vi "myRIO Main v2.vi"() -> ()   [LabVIEW 2014]
uses:
  Sensors/IMU - Adafruit BNO055/IMU Control.ctl
  <vilib>/Utility/RT CPU Load.ctl
  Sensors/Time of Flight - VL6180/VL6180 states.ctl
  <vilib>/Platform/TimedLoop/XDataNode/timing_clust.ctl
  <vilib>/Platform/TimedLoop/XDataNode/nitl_modes.ctl
  <vilib>/Platform/TimedLoop/XDataNode/wakeup.ctl
  <vilib>/myRIO/Instrument Drivers/Onboard IO/DIO/typedefs/DIO Reference.ctl
  <vilib>/myRIO/Common/Instrument Driver Framework/Utilities/typedefs/myRIO Generic Hardware Reference.ctl
  <vilib>/myRIO/Common/Instrument Driver Framework/Utilities/typedefs/Hardware Version Enum.ctl
  <vilib>/myRIO/Common/Instrument Driver Framework/Utilities/typedefs/myRIO v1.0 Reference.ctl
  <vilib>/myRIO/Common/Instrument Driver Framework/Utilities/typedefs/Generic FPGA Reference.ctl
  <vilib>/myRIO/Common/Instrument Driver Framework/myRIO v1.0/DIO/typedefs/DIO Channels List.ctl
  <vilib>/myRIO/Common/Instrument Driver Framework/myRIO v1.0/DIO/typedefs/DIO Channels Enum.ctl
  <vilib>/userdefined/High Color/nirio_resource_hc.ctl
  Sensors/Time of Flight - VL6180/VL6180 Resource.ctl
  <vilib>/myRIO/Common/Instrument Driver Framework/Utilities/vis/Is FPGA Ref Available.vi
  <vilib>/myRIO/Common/Instrument Driver Framework/myRIO v1.0/DIO/vis/myRIO v1.1 Open DIO.vi
  <vilib>/myRIO/Instrument Drivers/Onboard IO/DIO/vis/Read.vi
  <vilib>/myRIO/Instrument Drivers/Onboard IO/DIO/vis/Write.vi
  <vilib>/MakerHub/LINX/Public/Peripherals/Digital/Digital Write 1 Chan.vi
  <vilib>/myRIO/Common/Instrument Driver Framework/Utilities/vis/Validate Channels.vi
  <vilib>/myRIO/Common/Instrument Driver Framework/myRIO v1.0/DIO/vis/myRIO v1.0 Reserve DIO.vi
  <vilib>/MakerHub/LINX/Public/Utilities/Check Channel.vi
  <vilib>/MakerHub/LINX/Public/Peripherals/Digital/Digital Write N Chans.vi
  <vilib>/myRIO/Common/Instrument Driver Framework/myRIO v1.0/Resource Manager/vis/myRIO v1.0 Reserve Channel List.vi
  <vilib>/myRIO/Common/Instrument Driver Framework/myRIO v1.0/DIO/vis/myRIO v1.0 Build MUX Configuration DIO.vi
  <vilib>/MakerHub/LINX/Private/Local IO/LinxDigitalWrite.vi
  <vilib>/myRIO/Common/Instrument Driver Framework/myRIO v1.0/Resource Manager/vis/myRIO v1.0 Reserve Channel.vi
  <vilib>/myRIO/Common/Instrument Driver Framework/myRIO v1.0/Resource Manager/vis/myRIO v1.0 Unreserve Channel.vi
  <vilib>/myRIO/Common/Instrument Driver Framework/myRIO v1.0/Resource Manager/vis/myRIO v1.0 Create Configuration List.vi
  <vilib>/MakerHub/LINX/Private/myRIO/Utilities/Get DIO Channel Name.vi
  <vilib>/myRIO/Common/Instrument Driver Framework/myRIO v1.0/Resource Manager/vis/myRIO v1.0 Build Mutex Name.vi
  <vilib>/MakerHub/LINX/Public/Utilities/Open Local.vi
  <vilib>/MakerHub/LINX/Private/Utilties/Generate Error.vi
  <vilib>/MakerHub/LINX/Private/Local IO/LinxI2cOpen.vi
  <vilib>/Utility/VariantDataType/GetNumericInfo.vi
  <vilib>/Utility/error.llb/Error Cluster From Error Code.vi
  <vilib>/myRIO/Common/Instrument Driver Framework/myRIO v1.0/myRIO v1.1 Open.vi
  <vilib>/myRIO/Common/Instrument Driver Framework/Utilities/vis/IO Manager.vi
  <vilib>/myRIO/Common/Instrument Driver Framework/Utilities/vis/Configuration Manager.vi
  <vilib>/myRIO/Common/Instrument Driver Framework/myRIO v1.0/Resource Manager/vis/myRIO v1.0 Configure IO.vi
  <vilib>/myRIO/Common/Instrument Driver Framework/myRIO v1.0/myRIO v1.0 Close.vi
  <vilib>/myRIO/Common/Instrument Driver Framework/myRIO v1.0/DIO/vis/myRIO v1.0 Write DIO.vi
  <vilib>/myRIO/Instrument Drivers/Onboard IO/DIO/vis/Smart Open.vi
  <vilib>/myRIO/Common/Instrument Driver Framework/myRIO v1.0/DIO/vis/myRIO v1.0 Read DIO.vi
  <vilib>/myRIO/Express VI/Onboard IO/DO/DO Express VI.xnode
  <vilib>/myRIO/Instrument Drivers/Onboard IO/DIO/vis/myRIO DIO Open.xnode
  <vilib>/platform/TimedLoop/XDataNode/XDataNode.xnode
  <vilib>/myRIO/Express VI/Onboard IO/DI/DI Express VI.xnode
  <vilib>/MakerHub/LINX/LMH-LINX.lvlib
  <vilib>/Platform/TimedLoop/XDataNode/XDNodeRunTimeDep.lvlib
  <vilib>/myRIO/Instrument Drivers/Onboard IO/DIO/DIO.lvlib
  <vilib>/NI_Real-Time Target Support.lvlib
panel:
  in  "stop":bool
  in  "Enqueue Element":bool
  out "CPU loads":T1[](array[typedef]) {"ISR (%)" format="%#.2f"; "Idle (%)" format="%#.2f"; "Background (%)" format="%#.2f"; "Normal (%)" format="%#.2f"; "Above Normal (%)" format="%#.2f"; "High (%)" format="%#.2g"; "Timed Structures (%)" format="%#.2g"; "Time Critical (%)" format="%#.2g"; "Total (%)" format="%#.2g"}
  out "Pod Health":cluster{"Urgency":u32, "Status":string}
  out "Conversion Time (S)":dbl format="%#_g s"
  out "Power":dbl(knob) scale=0.0..10.0
  out "Current":dbl(knob) scale=0.0..2.0
  out "Voltage":dbl(knob) scale=11.0..12.0
  out "Pressure":i32(graph)
  out "Temp1":dbl(slide) scale=0.0..100.0
  out "V & P Monitor":cluster{"Voltage (Total)":dbl, "Power":dbl}(graph)
  in  "Sensor Power":bool=TRUE
  out "Laser Error":bool
  in  "Reset":bool
  in  "Stop":bool
  in  "Wait (ms)":u32=10
  out "ToF Loop Rate":u32
  in  "Speed Read":bool
  out "Attempts":i32
  out "Sensor Error Code":u8
  in  "Attempts before Timeout":u16=10
  in  "delay":u32=100
  in  "I2C Channel":u8
  out "Sensors Online":bool[](array[boolean])
  in  "# of sensors":i32=5
  out "Status":string
  in  "Track Location":dbl(slide) scale=0.0..5000.0
  out "Structure\nStress":dbl(slide) scale=2.4..2.6
  out "Track Position":T2
  out "Battery (Primary)":dbl(slide) scale=0.0..100.0 scale format="%.1f%"
  out "IMU":T3 {"Gyroscope"."Z" scale=-45.0..45.0; "Gyroscope"."Y" scale=-45.0..45.0; "Gyroscope"."X" scale=-45.0..45.0; "Magnetometer"."Z" scale=-2500.0..2500.0; "Magnetometer"."Y" scale=-2500.0..2500.0; "Magnetometer"."X" scale=-2500.0..2500.0; "Accelerometer"."Z" scale=-5.0..5.0; "Accelerometer"."Y" scale=-5.0..5.0; "Accelerometer"."X" scale=-5.0..5.0}
  out "Gap 4":u8(slide) scale=0.0..100.0
  out "Gap 3":u8(slide) scale=0.0..200.0
  out "Rail Gap 2":u8(slide) scale=0.0..100.0
  out "Gap 2":u8(slide) scale=0.0..100.0
  out "Temp 2":dbl(slide) scale=0.0..100.0
  out "Rail Gap 1":u8(slide) scale=0.0..100.0
  out "Gap 1":u8(slide) scale=0.0..100.0
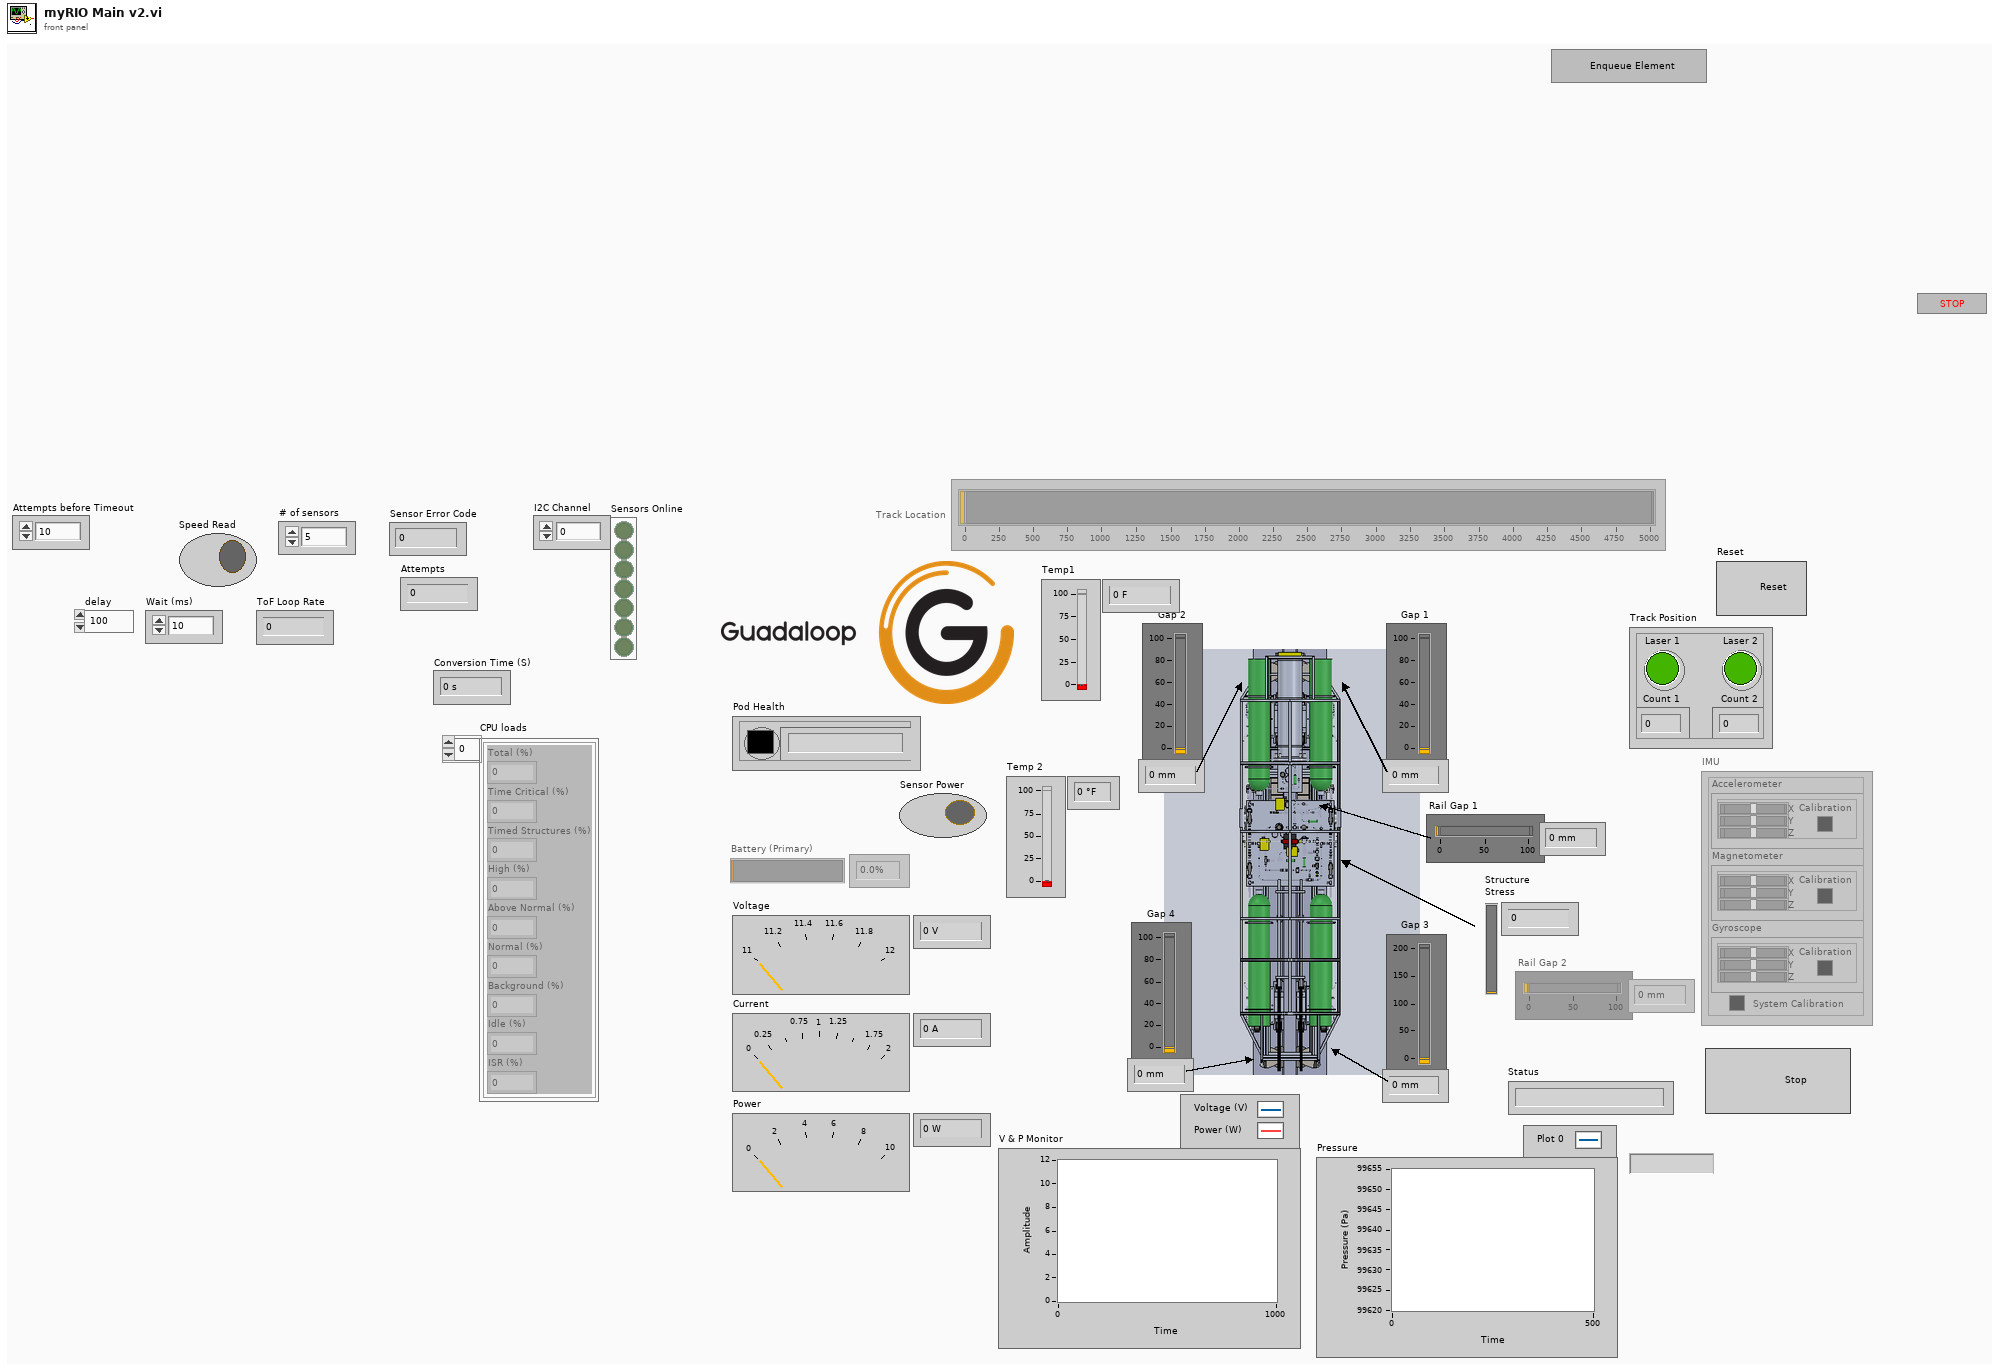
[diagram p1: front panel]
types:
  T1 = typedef "NI_Real-Time Target Support.lvlib/RT CPU Load.ctl" = cluster{"Total (%)":dbl, "Time Critical (%)":dbl, "Timed Structures (%)":dbl, "High (%)":dbl, "Above Normal (%)":dbl, "Normal (%)":dbl, "Background (%)":dbl, "Idle (%)":dbl, "ISR (%)":dbl}
  T2 = cluster{"Laser 1":bool, "Count 1":u32, "Laser 2":bool, "Count 2":u32}
  T3 = typedef "IMU Control.ctl" = cluster{"Accelerometer":cluster{"X":dbl, "Y":dbl, "Z":dbl, "Calibration":u32}, "Magnetometer":cluster{"X":dbl, "Y":dbl, "Z":dbl, "Calibration":u32}, "Gyroscope":cluster{"X":dbl, "Y":dbl, "Z":dbl, "Calibration":u32}, "System Calibration":u32}
  T4 = typedef "VL6180 states.ctl" = enum16{"Ping All", "Initialize", "Read"}
  T5 = typedef "LMH-LINX.lvlib/LINX Ref.ctl" = cluster{"IO":T6, "Interface":T7, "LINX Device Config":T8}
  T6 = typedef "LMH-LINX.lvlib/Platform.ctl" = enum16{"Remote", "Local"}
  T7 = typedef "LMH-LINX.lvlib/Interface.ctl" = enum16{"Serial", "TCP"}
  T8 = typedef "LMH-LINX.lvlib/Device.lvlib/LINX Device Config.ctl" = cluster{"Interface":T7, "COM Port":refnum<visa-resource-name>, "TCP Configuration":T9, "Device Family":u8, "Device ID":u8, "Device Name":string, "TCP Ref":refnum<k5>, "Channels":T10}
  T9 = typedef "LMH-LINX.lvlib/Device.lvlib/TCP Config.ctl" = cluster{"IP Address":string, "Port":u16}
  T10 = typedef "LMH-LINX.lvlib/Channels.ctl" = cluster{"DI":u8[], "DO":u8[], "AI":u8[], "AO":u8[], "PWM":u8[], "QE":u8[], "UART":u8[], "I2C 2":u8[], "SPI":u8[], "CAN":u8[], "Servo":u8[], "AI Ref (V)":dbl, "AI Resolution (Bits)":u8, "AO Ref (V)":dbl, "AO Resolution (Bits)":u8}
  T11 = typedef "XDNodeRunTimeDep.lvlib/timing_clust.ctl" = cluster{"Expected End [f-1]":u64, "Actual End [f-1]":u64, "Finished Late? [f-1]":bool, "Expected End [i-1]":u64, "Actual End [i-1]":u64, "Finished Late? [i-1]":bool, "Expected Start [i]":u64, "Actual Start [i]":u64, "Expected Start [f]":u64, "Actual Start [f]":u64, "Source Name":string, "Structure Name":string, "Period":i64, "Deadline":i64, "Offset":i64, "Start":i64, "Priority":i32, "Timeout":i32, "Mode":T12, "Wakeup Reason":T13, "Error":errorcluster, "Source Type":string, "Secondary Source Type":string, "Global End Time":u64, "Global Start Time":u64, "Frame Duration":u64, "Iteration Duration":u64, "Assigned CPU":i32, "I/O Scan Engine Mode":u32}
  T12 = typedef "XDNodeRunTimeDep.lvlib/nitl_modes.ctl" = enum32{"No Change", "Process missed periods, maintain original phase", "Discard missed periods, maintain original phase", "Process missed periods, ignore original phase", "Discard missed periods, ignore original phase"}
  T13 = typedef "XDNodeRunTimeDep.lvlib/wakeup.ctl" = enum32{"Normal", "Aborted", "Asynchronous wakeup", "Timing source error", "Timed loop error", "Timeout"}
  T14 = typedef "DIO.lvlib/DIO Reference.ctl" = cluster{"myRIO Reference":T15, "DIO Channels List":T19}
  T15 = typedef "myRIO Generic Hardware Reference.ctl" = cluster{"myRIO Model":T16, "myRIO Hardware Reference":T17}
  T16 = typedef "Hardware Version Enum.ctl" = enum16{"Unknown", "myRIO-1900", "myRIO-1950"}
  T17 = typedef "myRIO v1.0 Reference.ctl" = cluster{"Generic FPGA Reference":T18, "Allow multiple opens":bool}
  T18 = typedef "Generic FPGA Reference.ctl" = refnum<k20>
  T19 = typedef "DIO Channels List.ctl" = T20[]
  T20 = typedef "DIO Channels Enum.ctl" = enum16{"Not Connected", "C/DIO0", "C/DIO1", "C/DIO2", "C/DIO3", "C/DIO4", "C/DIO5", "C/DIO6", "C/DIO7", "A/DIO0", "A/DIO1", "A/DIO2", "A/DIO3", "A/DIO4", "A/DIO5", "A/DIO6", "A/DIO7", "A/DIO8", "A/DIO9", "A/DIO10", "A/DIO11", "A/DIO12", "A/DIO13", "A/DIO14", "A/DIO15", "B/DIO0", "B/DIO1", "B/DIO2", "B/DIO3", "B/DIO4", "B/DIO5", "B/DIO6", "B/DIO7", "B/DIO8", "B/DIO9", "B/DIO10", "B/DIO11", "B/DIO12", "B/DIO13", "B/DIO14", "B/DIO15", "LED0", "LED1", "LED2", "LED3", "Button0"}
  T21 = typedef "nirio_resource_hc.ctl" = tag
  T22 = typedef "VL6180 Resource.ctl" = cluster{"I2C Channel":u8, "I2C Slave Address":u8, "Online":bool}
  T23 = cluster{"Object Temp (°C)":dbl, "Object Temp (°F)":dbl, "Ambient Temp (°C)":dbl, "Ambient Temp (°F)":dbl}
  T24 = typedef "INA219 Measurements.ctl" = cluster{"Voltage (Total)":dbl, "Bus Voltage":dbl, "Shunt Voltage":dbl, "Power":dbl, "Current":dbl}
  T25 = typedef "INA219 Config Options.ctl" = cluster{"I2C":cluster{"Slave Address":u8, "Channel":u8}, "Reset bit":u8, "Bus Voltage Range":u8, "PGA/Shunt Voltage Gain":u8, "Bus Voltage ADC Settings":u8, "Shunt Voltage ADC Settings":u8, "Mode":u8, "Calibration Value":u16}
  T26 = typedef "BMP180 Config Options.ctl" = cluster{"I2C":cluster{"Slave Address":u8, "Channel":u8}, "Mode":enum8{"Ultra Low Power", "Standard", "High Resolution", "Ultra High Resolution"}, "Cal Coefs":cluster{"AC1":cluster{"Addr:":u8, "Val:":u16}, "AC2":cluster{"Addr:":u8, "Val:":u16}, "AC3":cluster{"Addr:":u8, "Val:":u16}, "AC4":cluster{"Addr:":u8, "Val:":u16}, "AC5":cluster{"Addr:":u8, "Val:":u16}, "AC6":cluster{"Addr:":u8, "Val:":u16}, "B1":cluster{"Addr:":u8, "Val:":u16}, "B2":cluster{"Addr:":u8, "Val:":u16}, "MB":cluster{"Addr:":u8, "Val:":u16}, "MC":cluster{"Addr:":u8, "Val:":u16}, "MD":cluster{"Addr:":u8, "Val:":u16}}}
  T27 = typedef "ADS1015 Config Options.ctl" = cluster{"I2C":cluster{"Slave Address":u8, "Channel":u8}, "ADC":cluster{"Channel":u8, "Expected Range (Programmable Gain Amplifier)":u8, "Sampling Mode":u8, "Sampling Rate":u8, "Comparator Mode":u8, "Comparator Polarity":u8, "Latching Comparator":u8, "Comparator Queue & Disable":u8}}
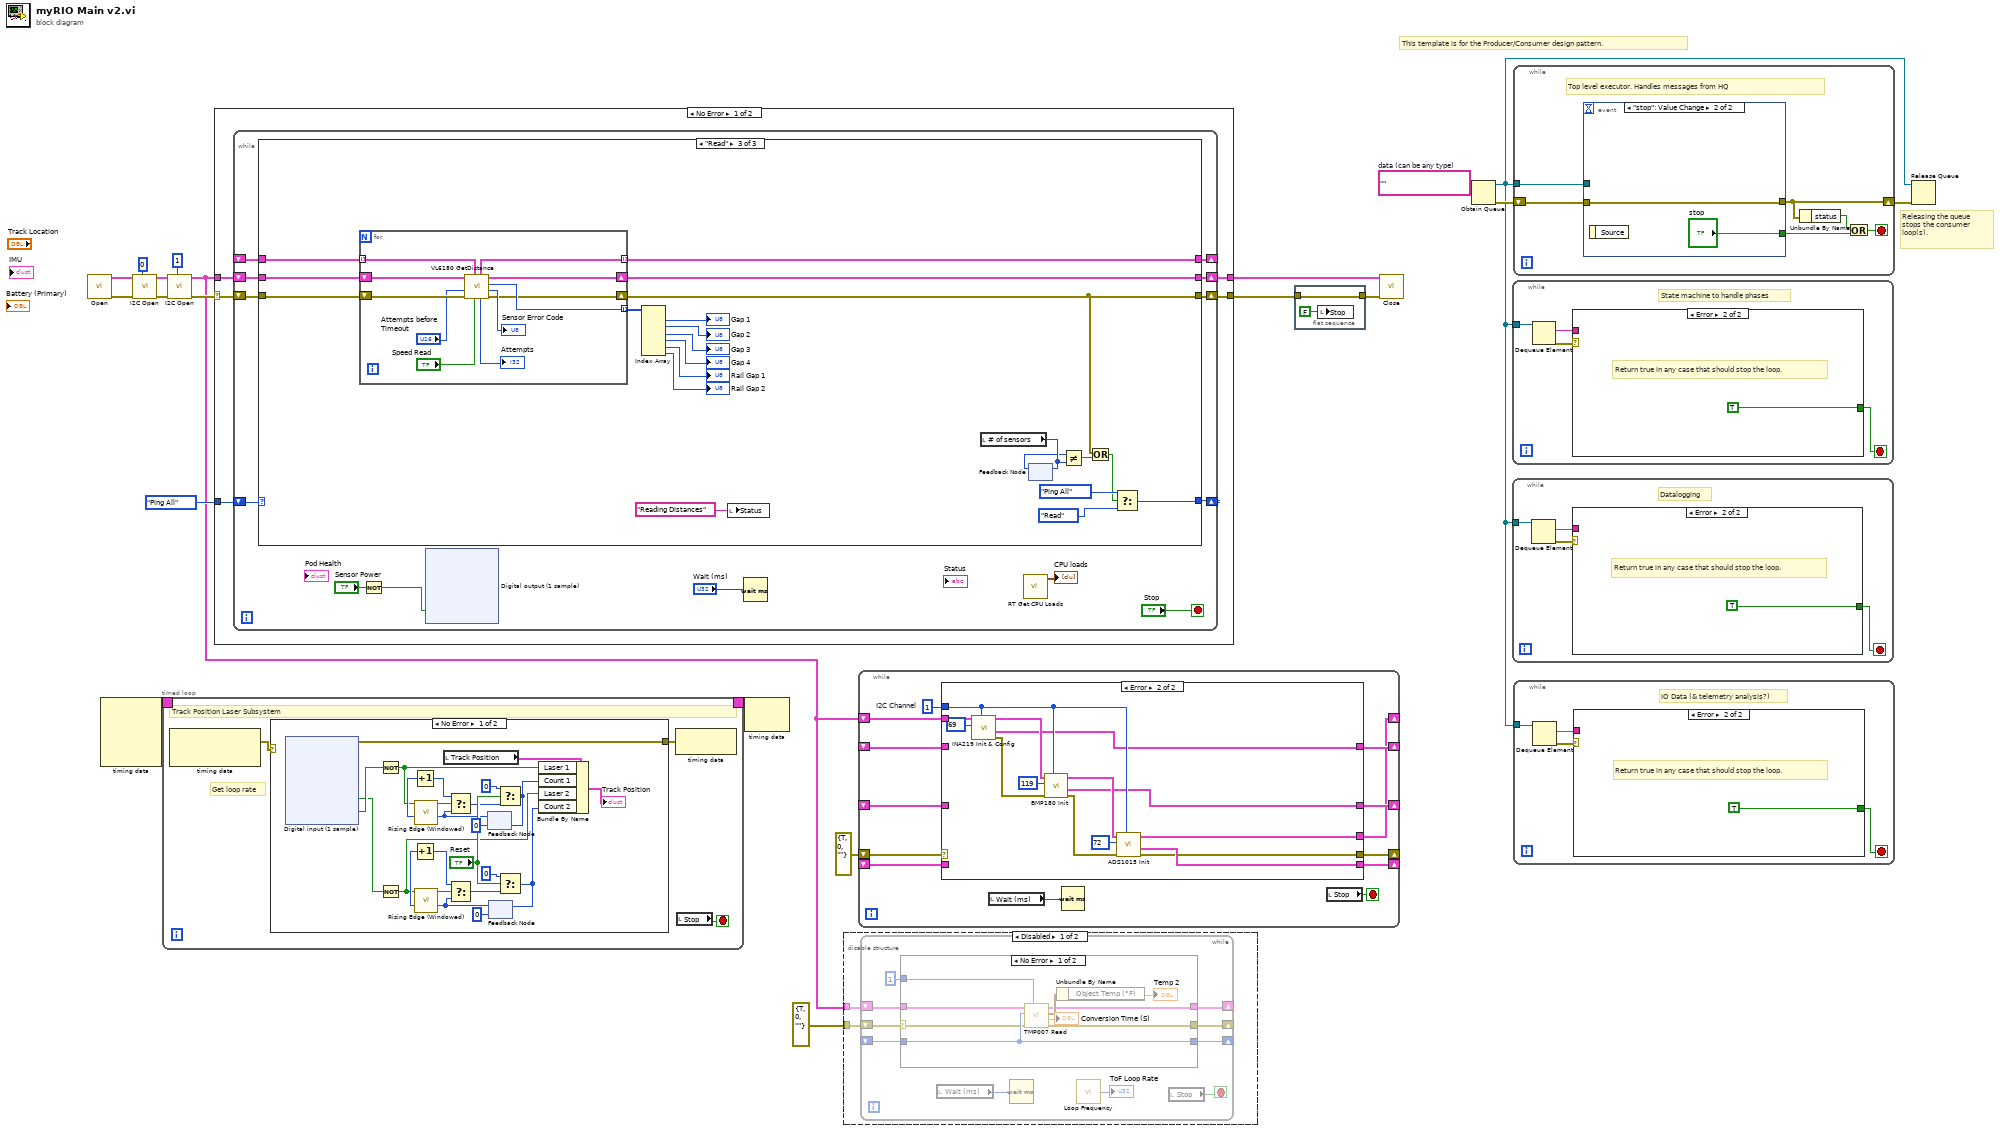
[diagram p0: block diagram]
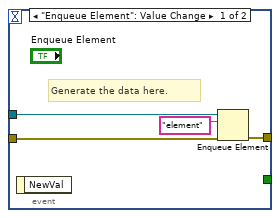
[diagram p5: hidden frame]
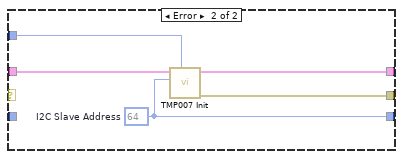
[diagram p6: hidden frame]
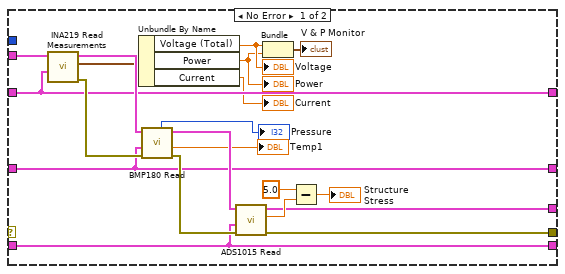
[diagram p8: hidden frame]
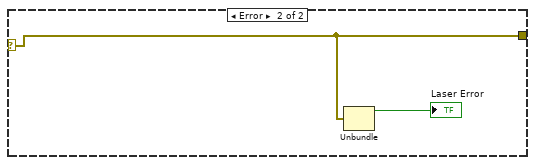
[diagram p9: hidden frame]
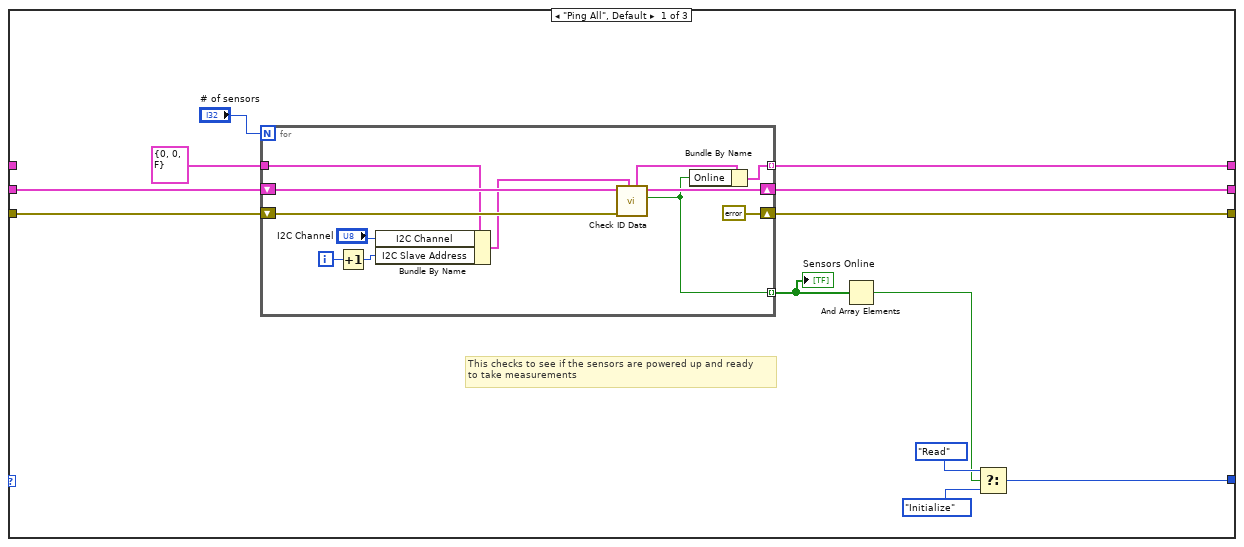
[diagram p10: hidden frame]
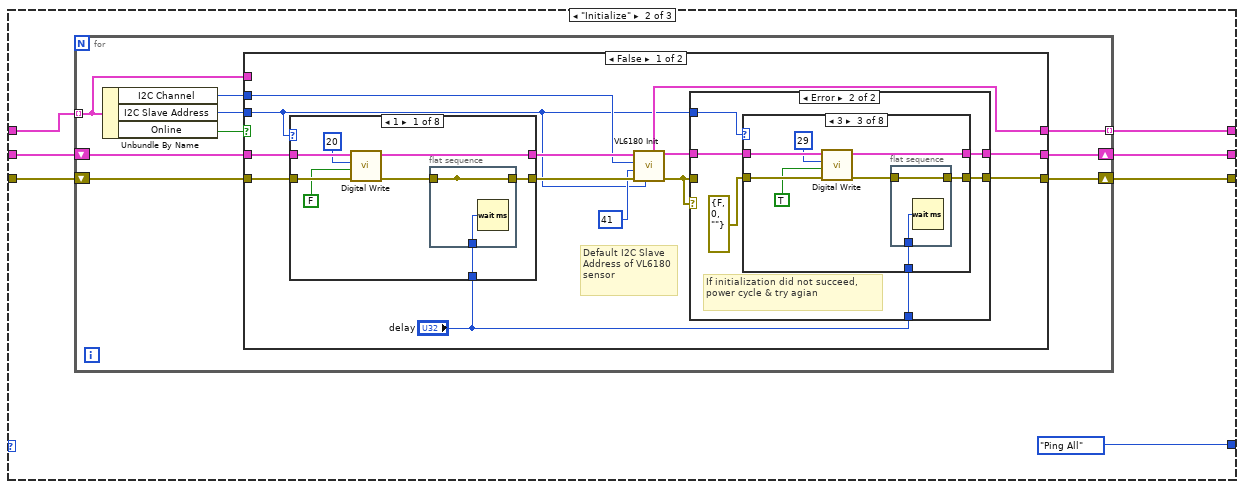
[diagram p11: hidden frame]
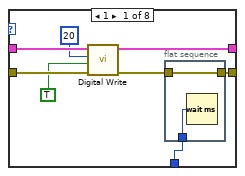
[diagram p13: hidden frame]
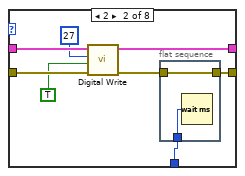
[diagram p14: hidden frame]
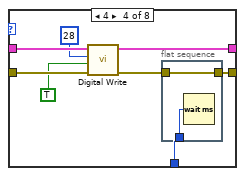
[diagram p15: hidden frame]
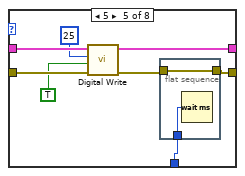
[diagram p16: hidden frame]
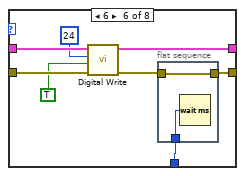
[diagram p17: hidden frame]
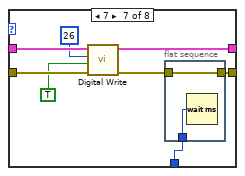
[diagram p18: hidden frame]
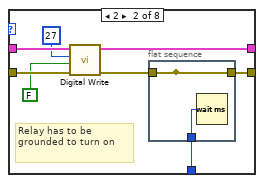
[diagram p20: hidden frame]
diagram:
  w2 = ""  # data (can be any type)
  # "Releasing the queue stops the consumer loop(s)."
  # "This template is for the Producer/Consumer design pattern."
  n1 = call-poly <vilib>:"Open.vi"() -> ("Error Out"=w10:errorcluster, "LINX Resource"=w11:T5)  [unwired: 9 in, 1 out]
  n2 = node-c288() -> (w16:T11)  [unwired: 4 in]
  n3 = call <vilib>:"I2C Open.vi"("I2C Channel (0)"=u8 0, "Error In"=w10, "LINX Resource"=w11) -> ("Error Out"=w9:errorcluster, "LINX Resource"=w8:T5)  [unwired: 7 in]
  n4 = timed-loop {
    timing: w16 -> [_]
    timing-out: [_] -> w15
    stop <- w23 stop-if-true
    # "Get loop rate"
    # "Track Position Laser Subsystem"
    n5 = node-c288() -> (w22:errorcluster)  [unwired: 1 in, 1 out]
    n6 = case shown="No Error" w22 {
      selector: w22 -> [_ w83]
      tunnel: [w28 w83] -> w21
      frame No Error {
        n7 = xnode "Digital input (1 sample)"() -> ("Laser 1 (A/DIO0 (Pin 11))"=w24:bool, "Laser 2 (A/DIO1 (Pin 13))"=w25:bool, "error out"=w28:errorcluster)  [unwired: 1 in]
        n8 = Not(x=w25) -> (.not. x?=w33:bool)
        n9 = Not(x=w24) -> (.not. x?=w30:bool)
        n10 = call "Rising Edge (Windowed).vi"("Input"=w33) -> ("Rising Edge?"=w38:bool)  [unwired: 10 in]
        n11 = call "Rising Edge (Windowed).vi"("Input"=w30) -> ("Rising Edge?"=w31:bool)  [unwired: 10 in]
        n12 = local read "Track Position"() -> (w35:T2)
        n13 = feedback #1(u32 0 ("t")) -> (w37:u32)
        n14 = Increment(x=w37) -> (x+1=w39:u32)
        n15 = Select(t=w39, s=w38, f=w37) -> (s? t:f=w40:u32)
        n16 = feedback #2(u32 0 ("t")) -> (w36:u32)
        n17 = Increment(x=w36) -> (x+1=w42:u32)
        n18 = Select(t=w42, s=w31, f=w36) -> (s? t:f=w43:u32)
        n19 = Select(t=u32 0, s="Reset", f=w40) -> (s? t:f=w32:u32)
        n20 = feedback-in #1(w32) -> ()
        n21 = Select(t=u32 0, s="Reset", f=w43) -> (s? t:f=w29:u32)
        n22 = feedback-in #2(w29) -> ()
        n23 = Bundle By Name(cluster=w35, "Laser 1"=w33, "Count 1"=w32, "Laser 2"=w30, "Count 2"=w29) -> (→"Track Position":T2)
      }
      frame Error {
        n24 = Unbundle(w83) -> ("status"=→"Laser Error":bool)  [unwired: 2 out]
      }
    }
    n25 = node-c288(w21) -> ()  [unwired: 1 out]
    n26 = local read "Stop"() -> (w23:bool)
  }
  n27 = call <vilib>:"I2C Open.vi"("I2C Channel (0)"=u8 1, "Error In"=w9, "LINX Resource"=w8) -> ("Error Out"=w14:errorcluster, "LINX Resource"=w5:T5)  [unwired: 7 in]
  n28 = case shown="No Error" w14 {
    selector: w14 -> [w91 w384]
    tunnel: [w93 w384] -> w18
    tunnel: [w92 w383] -> w19
    tunnel: VL6180_states."Ping All" -> [w90 _]
    tunnel: w5 -> [w89 w383]
    frame No Error {
      n29 = while {
        shift-right: [w98] -> w92
        shift-left: w89 -> [w104]
        shift-right: [w97] -> w93
        shift-left: w91 -> [w103]
        shift-right: [w99] -> _
        shift-left: _ -> [w102]
        shift-right: [w100] -> _
        shift-left: w90 -> [w101]
        stop <- "Stop" stop-if-true
        n30 = case shown="\"Read\"" w101 {
          tunnel: w104 -> [w118 w137 w334]
          tunnel: w103 -> [w117 w131 w336]
          tunnel: w102 -> [_ w135 w333]
          tunnel: [w115 w132 w335] -> w99
          tunnel: [w116 w134 w328] -> w98
          tunnel: [w114 VL6180_states."Ping All" w332] -> w100
          tunnel: [w113 w133 w327] -> w97
          frame "Ping All", Default {
            # "This checks to see if the sensors are powered up and ready\nto take measurements"
            n31 = for {
              N: "# of sensors" -> [_]
              tunnel: T22 {"I2C Channel"=0, "I2C Slave Address"=0, "Online"=FALSE} ("VL6180 Resource out") -> [w123]
              shift-right: [w126] -> w116
              shift-left: w118 -> [w130]
              tunnel: [w125] -> w115 mode=indexing
              tunnel: [w124] -> w112 mode=indexing
              shift-right: [errorcluster {"status"=FALSE, "code"=0, "source"=""} ("error IO")] -> w113
              shift-left: w117 -> [w129]
              i -> [w127]
              n32 = Increment(x=w127) -> (x+1=w120:i32)
              n33 = Bundle By Name(cluster=w123, "I2C Channel"="I2C Channel", "I2C Slave Address"=w120) -> (w122:T22)
              n34 = call "Check ID Data.vi"("VL6180 Resource"=w122, "Error In"=w129, "LINX Resource"=w130) -> ("Same Model?"=w124:bool, "LINX Resource"=w126:T5, "VL6180 Resource"=w128:T22)  [unwired: 5 in, 1 out]
              n35 = Bundle By Name(cluster=w128, "Online"=w124) -> (w125:T22)
            }
            "Sensors Online" <- w112
            n36 = And Array Elements(Boolean array=w112) -> (logical AND=w109:bool)
            n37 = Select(t=VL6180_states."Read", s=w109, f=VL6180_states."Initialize") -> (s? t:f=w114:T4)
          }
          frame "Initialize" {
            n38 = for {
              tunnel: w135 -> [w138] mode=indexing
              shift-right: [w145] -> w134
              shift-left: w137 -> [w146]
              shift-right: [w144] -> w133
              shift-left: w131 -> [w140]
              tunnel: [w141] -> w132 mode=indexing
              n39 = Unbundle By Name(w138) -> ("I2C Channel"=w143:u8, "I2C Slave Address"=w142:u8, "Online"=w139:bool)
              n40 = case shown="False" w139 {
                tunnel: w146 -> [w159 w315]
                tunnel: w140 -> [w156 w314]
                tunnel: [w153 w315] -> w145
                tunnel: [w152 w314] -> w144
                tunnel: w143 -> [w148 _]
                tunnel: w142 -> [w147 _]
                tunnel: [w154 w313] -> w141
                tunnel: w138 -> [_ w313]
                frame False {
                  # "Default I2C Slave Address of VL6180 sensor"
                  n41 = case shown="1" w147 {
                    tunnel: w159 -> [w247 w257 w267 w277 w287 w297 w307 w311]
                    tunnel: [w246 w256 w266 w276 w286 w296 w306 w311] -> w158
                    tunnel: [w242 w252 w261 w271 w281 w291 w301 w310] -> w157
                    tunnel: w156 -> [w245 w255 w265 w275 w285 w295 w305 w310]
                    tunnel: "delay" -> [w240 w250 w260 w270 w280 w290 w300 _]
                    frame 1 {
                      n42 = call-poly <vilib>:"Digital Write.vi"("Error In"=w245, "Output Value"=FALSE, "DO Channel"=u8 20, "LINX Resource"=w247) -> ("Error Out"=w241:errorcluster, "LINX Resource"=w246:T5)  [unwired: 6 in]
                      n43 = flat-sequence {
                        tunnel: [w249] -> _
                        tunnel: [w249] -> w242
                        tunnel: w241 -> [w249]
                        tunnel: w240 -> [w248]
                        frame #0 {
                          n44 = Wait (ms)(milliseconds to wait=w248) -> ()  [unwired: 1 out]
                        }
                      }
                    }
                    frame 2 {
                      # "Relay has to be grounded to turn on"
                      n45 = call-poly <vilib>:"Digital Write.vi"("Error In"=w255, "Output Value"=FALSE, "DO Channel"=u8 27, "LINX Resource"=w257) -> ("Error Out"=w251:errorcluster, "LINX Resource"=w256:T5)  [unwired: 6 in]
                      n46 = flat-sequence {
                        tunnel: [w259] -> _
                        tunnel: [w259] -> w252
                        tunnel: w251 -> [w259]
                        tunnel: w250 -> [w258]
                        frame #0 {
                          n47 = Wait (ms)(milliseconds to wait=w258) -> ()  [unwired: 1 out]
                        }
                      }
                    }
                    frame 3 {
                      n48 = call-poly <vilib>:"Digital Write.vi"("Error In"=w265, "Output Value"=FALSE, "DO Channel"=u8 29, "LINX Resource"=w267) -> ("Error Out"=w262:errorcluster, "LINX Resource"=w266:T5)  [unwired: 6 in]
                      n49 = flat-sequence {
                        tunnel: w262 -> [w269]
                        tunnel: [w269] -> w261
                        tunnel: w260 -> [w268]
                        frame #0 {
                          n50 = Wait (ms)(milliseconds to wait=w268) -> ()  [unwired: 1 out]
                        }
                      }
                    }
                    frame 4 {
                      n51 = call-poly <vilib>:"Digital Write.vi"("Error In"=w275, "Output Value"=FALSE, "DO Channel"=u8 28, "LINX Resource"=w277) -> ("Error Out"=w272:errorcluster, "LINX Resource"=w276:T5)  [unwired: 6 in]
                      n52 = flat-sequence {
                        tunnel: w272 -> [w279]
                        tunnel: [w279] -> w271
                        tunnel: w270 -> [w278]
                        frame #0 {
                          n53 = Wait (ms)(milliseconds to wait=w278) -> ()  [unwired: 1 out]
                        }
                      }
                    }
                    frame 5 {
                      n54 = call-poly <vilib>:"Digital Write.vi"("Error In"=w285, "Output Value"=FALSE, "DO Channel"=u8 25, "LINX Resource"=w287) -> ("Error Out"=w282:errorcluster, "LINX Resource"=w286:T5)  [unwired: 6 in]
                      n55 = flat-sequence {
                        tunnel: w282 -> [w289]
                        tunnel: [w289] -> w281
                        tunnel: w280 -> [w288]
                        frame #0 {
                          n56 = Wait (ms)(milliseconds to wait=w288) -> ()  [unwired: 1 out]
                        }
                      }
                    }
                    frame 6 {
                      n57 = call-poly <vilib>:"Digital Write.vi"("Error In"=w295, "Output Value"=FALSE, "DO Channel"=u8 24, "LINX Resource"=w297) -> ("Error Out"=w292:errorcluster, "LINX Resource"=w296:T5)  [unwired: 6 in]
                      n58 = flat-sequence {
                        tunnel: w292 -> [w299]
                        tunnel: [w299] -> w291
                        tunnel: w290 -> [w298]
                        frame #0 {
                          n59 = Wait (ms)(milliseconds to wait=w298) -> ()  [unwired: 1 out]
                        }
                      }
                    }
                    frame 7 {
                      n60 = call-poly <vilib>:"Digital Write.vi"("Error In"=w305, "Output Value"=FALSE, "DO Channel"=u8 30, "LINX Resource"=w307) -> ("Error Out"=w302:errorcluster, "LINX Resource"=w306:T5)  [unwired: 6 in]
                      n61 = flat-sequence {
                        tunnel: w302 -> [w309]
                        tunnel: [w309] -> w301
                        tunnel: w300 -> [w308]
                        frame #0 {
                          n62 = Wait (ms)(milliseconds to wait=w308) -> ()  [unwired: 1 out]
                        }
                      }
                    }
                    frame 9, Default {
                      n63 = local write "Status"("Plug new sensor in" ("message")) -> ()
                    }
                  }
                  n64 = call "VL6180 Init.vi"("Change Slave Address"=w147, "Error In"=w157, "I2C Slave Address"=u8 41 ("I2C Slave Address (0)"), "I2C Channel"=w148, "LINX Resource"=w158) -> ("Error Out"=w150:errorcluster, "LINX Resource"=w151:T5, "VL6180 Resource"=w154:T22)  [unwired: 4 in]
                  n65 = case shown="Error" w150 {
                    tunnel: [w161 w167] -> w153
                    tunnel: [w160 w164] -> w152
                    tunnel: w151 -> [w161 w166]
                    tunnel: w150 -> [w160 _]
                    tunnel: "delay" -> [_ w163]
                    tunnel: w147 -> [_ w162]
                    frame No Error {
                      # "Initialization successful"
                    }
                    frame Error {
                      # "If initialization did not succeed, power cycle & try agian"
                      n66 = case shown="3" w162 {
                        tunnel: w166 -> [w175 w185 w195 w205 w215 w225 w235 w239]
                        tunnel: [w174 w184 w194 w204 w214 w224 w234 w239] -> w167
                        tunnel: [w169 w178 w189 w199 w209 w219 w229 w238] -> w164
                        tunnel: errorcluster {"status"=FALSE, "code"=0, "source"=""} ("Error Out") -> [w173 w183 w193 w203 w213 w223 w233 w238]
                        tunnel: w163 -> [w168 w179 w188 w198 w208 w218 w228 _]
                        frame 1 {
                          n67 = call-poly <vilib>:"Digital Write.vi"("Error In"=w173, "Output Value"=TRUE, "DO Channel"=u8 20, "LINX Resource"=w175) -> ("Error Out"=w170:errorcluster, "LINX Resource"=w174:T5)  [unwired: 6 in]
                          n68 = flat-sequence {
                            tunnel: [w177] -> w169
                            tunnel: w170 -> [w177]
                            tunnel: w168 -> [w176]
                            frame #0 {
                              n69 = Wait (ms)(milliseconds to wait=w176) -> ()  [unwired: 1 out]
                            }
                          }
                        }
                        frame 2 {
                          n70 = call-poly <vilib>:"Digital Write.vi"("Error In"=w183, "Output Value"=TRUE, "DO Channel"=u8 27, "LINX Resource"=w185) -> ("Error Out"=w180:errorcluster, "LINX Resource"=w184:T5)  [unwired: 6 in]
                          n71 = flat-sequence {
                            tunnel: [w187] -> w178
                            tunnel: w180 -> [w187]
                            tunnel: w179 -> [w186]
                            frame #0 {
                              n72 = Wait (ms)(milliseconds to wait=w186) -> ()  [unwired: 1 out]
                            }
                          }
                        }
                        frame 3 {
                          n73 = call-poly <vilib>:"Digital Write.vi"("Error In"=w193, "Output Value"=TRUE, "DO Channel"=u8 29, "LINX Resource"=w195) -> ("Error Out"=w190:errorcluster, "LINX Resource"=w194:T5)  [unwired: 6 in]
                          n74 = flat-sequence {
                            tunnel: [w197] -> w189
                            tunnel: w190 -> [w197]
                            tunnel: w188 -> [w196]
                            frame #0 {
                              n75 = Wait (ms)(milliseconds to wait=w196) -> ()  [unwired: 1 out]
                            }
                          }
                        }
                        frame 4 {
                          n76 = call-poly <vilib>:"Digital Write.vi"("Error In"=w203, "Output Value"=TRUE, "DO Channel"=u8 28, "LINX Resource"=w205) -> ("Error Out"=w200:errorcluster, "LINX Resource"=w204:T5)  [unwired: 6 in]
                          n77 = flat-sequence {
                            tunnel: [w207] -> w199
                            tunnel: w200 -> [w207]
                            tunnel: w198 -> [w206]
                            frame #0 {
                              n78 = Wait (ms)(milliseconds to wait=w206) -> ()  [unwired: 1 out]
                            }
                          }
                        }
                        frame 5 {
                          n79 = call-poly <vilib>:"Digital Write.vi"("Error In"=w213, "Output Value"=TRUE, "DO Channel"=u8 25, "LINX Resource"=w215) -> ("Error Out"=w210:errorcluster, "LINX Resource"=w214:T5)  [unwired: 6 in]
                          n80 = flat-sequence {
                            tunnel: [w217] -> w209
                            tunnel: w210 -> [w217]
                            tunnel: w208 -> [w216]
                            frame #0 {
                              n81 = Wait (ms)(milliseconds to wait=w216) -> ()  [unwired: 1 out]
                            }
                          }
                        }
                        frame 6 {
                          n82 = call-poly <vilib>:"Digital Write.vi"("Error In"=w223, "Output Value"=TRUE, "DO Channel"=u8 24, "LINX Resource"=w225) -> ("Error Out"=w220:errorcluster, "LINX Resource"=w224:T5)  [unwired: 6 in]
                          n83 = flat-sequence {
                            tunnel: [w227] -> w219
                            tunnel: w220 -> [w227]
                            tunnel: w218 -> [w226]
                            frame #0 {
                              n84 = Wait (ms)(milliseconds to wait=w226) -> ()  [unwired: 1 out]
                            }
                          }
                        }
                        frame 7 {
                          n85 = call-poly <vilib>:"Digital Write.vi"("Error In"=w233, "Output Value"=TRUE, "DO Channel"=u8 26, "LINX Resource"=w235) -> ("Error Out"=w230:errorcluster, "LINX Resource"=w234:T5)  [unwired: 6 in]
                          n86 = flat-sequence {
                            tunnel: [w237] -> w229
                            tunnel: w230 -> [w237]
                            tunnel: w228 -> [w236]
                            frame #0 {
                              n87 = Wait (ms)(milliseconds to wait=w236) -> ()  [unwired: 1 out]
                            }
                          }
                        }
                        frame 9, Default {
                        }
                      }
                    }
                  }
                }
                frame True {
                }
              }
            }
          }
          frame "Read" {
            n88 = for {
              tunnel: [w343] -> w335 mode=indexing
              shift-right: [w341] -> w328
              shift-left: w334 -> [w342]
              tunnel: w333 -> [w337] mode=indexing
              tunnel: [w340] -> w321 mode=indexing
              shift-right: [w339] -> w327
              shift-left: w336 -> [w347]
              n89 = call "VL6180 GetDistance.vi"("Speed Read"="Speed Read", "VL6180 Resource in"=w337, "error in (no error)"=w347, "Attempts before Timeout"="Attempts before Timeout", "LINX Resource"=w342) -> ("error out"=w339:errorcluster, "Sensor Error Code"=→"Sensor Error Code":u8, "Distance (mm)"=w340:u8, "LINX Resource"=w341:T5, "Attempts"=→"Attempts":i32, "VL6180 Resource out"=w343:T22)  [unwired: 1 in]
            }
            n90 = Index Array(array=w321) -> (element #1=→"Gap 1":u8, element #2=→"Gap 2":u8, element #3=→"Gap 3":u8, element #4=→"Gap 4":u8, element #5=→"Rail Gap 1":u8, element #6=→"Rail Gap 2":u8)  [unwired: 6 in]
            n91 = local write "Status"("Reading Distances" ("Status")) -> ()
            n92 = local read "# of sensors"() -> (w325:i32)
            n93 = feedback-in #3(w325) -> ()
            n94 = feedback #3() -> (w324:i32)  [unwired: 1 in]
            n95 = Not Equal?(x=w324, y=w325) -> (x != y?=w326:bool)
            n96 = Or(x=w327, y=w326) -> (x .or. y?=w323:bool)
            n97 = Select(t=VL6180_states."Ping All", s=w323, f=VL6180_states."Read") -> (s? t:f=w332:T4)
          }
        }
        n98 = Not(x="Sensor Power") -> (.not. x?=w95:bool)
        n99 = xnode "Digital output (1 sample)"("Sens. Pow. (B/DIO7 (Pin 25))"=w95) -> ()  [unwired: 1 in, 1 out]
        n100 = Wait (ms)(milliseconds to wait="Wait (ms)") -> ()  [unwired: 1 out]
        n101 = call <vilib>:"RT Get CPU Loads.vi"() -> ("CPU loads"=→"CPU loads":T1[])  [unwired: 10 in, 1 out]
      }
    }
    frame Error {
    }
  }
  n102 = node-c288(w15) -> ()  [unwired: 1 out]
  n103 = disable-structure shown="Disabled" {
    disable-tunnel: errorcluster {"status"=TRUE, "code"=0, "source"=""} ("error out") -> [w386 _]
    disable-tunnel: w5 -> [w385 _]
    frame Disabled {
      n104 = while {
        shift-right: [w395] -> _
        shift-left: w386 -> [w394]
        shift-right: [w393] -> _
        shift-left: _ -> [w392]
        shift-right: [w389] -> _
        shift-left: w385 -> [w388]
        stop <- w396 stop-if-true
        n105 = case shown="No Error" w394 {
          selector: w394 -> [w399 _]
          tunnel: u8 1 ("I2C Channel") -> [w401 w407]
          tunnel: [w405 w410] -> w395
          tunnel: [w404 w409] -> w393
          tunnel: w392 -> [w404 _]
          tunnel: [w402 w408] -> w389
          tunnel: w388 -> [w398 w406]
          frame No Error {
            n106 = call "TMP007 Read.vi"("I2C Channel"=w401, "error in (no error)"=w399, "I2C Slave Address"=w404, "LINX Resource in"=w398) -> ("error out"=w405:errorcluster, "Conversion Time (S)"=→"Conversion Time (S)":dbl, "Temp Readings"=w403:T23, "LINX Resource"=w402:T5)  [unwired: 4 in]
            n107 = Unbundle By Name(w403) -> ("Object Temp (°F)"=→"Temp 2":dbl)
          }
          frame Error {
            w409 = u8 64  # I2C Slave Address
            n108 = call "TMP007 Init.vi"("I2C Channel"=w407, "I2C Slave Address"=w409, "LINX Resource in"=w406) -> ("error out"=w410:errorcluster, "LINX Resource out"=w408:T5)  [unwired: 7 in]
          }
        }
        n109 = local read "Wait (ms)"() -> (w391:u32)
        n110 = Wait (ms)(milliseconds to wait=w391) -> ()  [unwired: 1 out]
        n111 = call <vilib>:"Loop Frequency.vi"() -> ("Loop Rate (Hz)"=→"ToF Loop Rate":u32)
        n112 = local read "Stop"() -> (w396:bool)
      }
    }
    frame Enabled {
    }
  }
  n113 = while {
    shift-right: [w420] -> _
    shift-left: errorcluster {"status"=TRUE, "code"=0, "source"=""} ("error out") -> [w419]
    shift-right: [w418] -> _
    shift-left: _ -> [w413]
    shift-right: [w417] -> _
    shift-left: _ -> [w414]
    shift-right: [w416] -> _
    shift-left: _ -> [w415]
    shift-right: [w412] -> _
    shift-left: w5 -> [w423]
    stop <- w421 stop-if-true
    w422 = u8 1  # I2C Channel
    n114 = case shown="Error" w419 {
      tunnel: w423 -> [w443 w457]
      tunnel: w422 -> [_ w452]
      tunnel: [w425 w445] -> w420
      tunnel: [w438 w451] -> w418
      tunnel: [w437 w450] -> w417
      tunnel: [w436 w449] -> w416
      tunnel: w415 -> [w436 _]
      tunnel: w414 -> [w437 _]
      tunnel: w413 -> [w438 _]
      tunnel: [w424 w444] -> w412
      frame No Error {
        n115 = call "INA219 Read Measurements.vi"("INA219 Config Options"=w436, "LINX Resource in"=w443) -> ("error out"=w439:errorcluster, "Measurements"=w431:T24, "LINX Resource"=w442:T5)  [unwired: 7 in]
        n116 = Unbundle By Name(w431) -> ("Voltage (Total)"=w434:dbl, "Power"=w433:dbl, "Current"=→"Current":dbl)
        "Voltage" <- w434
        "Power" <- w433
        n117 = call "BMP180 Read.vi"("error in (no error)"=w439, "BMP180 Config"=w437, "LINX Resource in"=w442) -> ("error out"=w440:errorcluster, "Temperature (F)"=→"Temp1":dbl, "LINX Resource"=w441:T5, "Pressure"=→"Pressure":i32)  [unwired: 4 in, 1 out]
        n118 = call "ADS1015 Read.vi"("error in (no error)"=w440, "ADS1015 Config Options"=w438, "LINX Resource in"=w441) -> ("error out"=w425:errorcluster, "Voltage"=w428:dbl, "LINX Resource"=w424:T5)  [unwired: 5 in, 1 out]
        n119 = Bundle("Voltage (Total)"=w434, "Power"=w433) -> (→"V & P Monitor":cluster{"Voltage (Total)":dbl, "Power":dbl})  [unwired: 1 in]
        n120 = Subtract(x=5.0, y=w428) -> (x-y=→"Structure\nStress":dbl)
      }
      frame Error {
        n121 = call "INA219 Init & Config.vi"("I2C Channel"=w452, "I2C Slave Address"=u8 69, "LINX Resource in"=w457) -> ("error out"=w453:errorcluster, "INA219 Config Options"=w449:T25, "LINX Resource out"=w456:T5)  [unwired: 6 in]
        n122 = call "BMP180 Init.vi"("I2C Channel"=w452, "error in (no error)"=w453, "I2C Slave Address"=u8 119, "LINX Resource in"=w456) -> ("error out"=w454:errorcluster, "BMP180 Config Options"=w450:T26, "LINX Resource out"=w455:T5)  [unwired: 5 in]
        n123 = call "ADS1015 Init.vi"("I2C Channel"=w452, "error in (no error)"=w454, "I2C Slave Address"=u8 72, "LINX Resource in"=w455) -> ("error out"=w445:errorcluster, "ADS1015 Config Options"=w451:T27, "LINX Resource out"=w444:T5)  [unwired: 5 in]
      }
    }
    n124 = local read "Wait (ms)"() -> (w411:u32)
    n125 = Wait (ms)(milliseconds to wait=w411) -> ()  [unwired: 1 out]
    n126 = local read "Stop"() -> (w421:bool)
  }
  n127 = flat-sequence {
    tunnel: w18 -> [w458]
    tunnel: [w458] -> w17
    frame #0 {
      n128 = local write "Stop"(FALSE ("Stop")) -> ()
    }
  }
  n129 = call <vilib>:"Close.vi"("Error In"=w17, "LINX Resource"=w19) -> ()  [unwired: 9 in, 1 out]
  n130 = Obtain Queue(element data type=w2) -> (queue out=w1:refnum<queue>, error out=w4:errorcluster)  [unwired: 4 in, 1 out]
  n131 = while {
    tunnel: w1 -> [w463]
    stop <- w460 stop-if-true
    # "Datalogging"
    n132 = Dequeue Element(queue=w463) -> (element=w461:string, error out=w462:errorcluster)  [unwired: 2 in, 2 out]
    n133 = case shown="Error" w462 {
      tunnel: w461 -> [_ _]
      tunnel: [_ TRUE] -> w460
      frame No Error {
        # "Process the data here."
      }
      frame Error {
        # "Return true in any case that should stop the loop."
      }
    }
  }
  n134 = while {
    tunnel: w1 -> [w468]
    stop <- w465 stop-if-true
    # "State machine to handle phases"
    n135 = Dequeue Element(queue=w468) -> (element=w466:string, error out=w467:errorcluster)  [unwired: 2 in, 2 out]
    n136 = case shown="Error" w467 {
      tunnel: w466 -> [_ _]
      tunnel: [_ TRUE] -> w465
      frame No Error {
        # "Process the data here."
      }
      frame Error {
        # "Return true in any case that should stop the loop."
      }
    }
  }
  n137 = while {
    shift-right: [w471] -> w3
    shift-left: w4 -> [w474]
    tunnel: w1 -> [w475]
    stop <- w472 stop-if-true
    # "Top level executor. Handles messages from HQ"
    n138 = event shown="[1] \"stop\": Value Change" {
      selector: _ -> [_ _]
      dyn-events: _ -> [_ _]
      timeout: _ -> [_ _]
      tunnel: w475 -> [w479 _]
      tunnel: w474 -> [w478 w480]
      tunnel: [w477 w480] -> w471
      tunnel: [_ "stop"] -> w473
      event "Enqueue Element": Value Change {
        # "Generate the data here."
        n139 = event-data() -> ()  [unwired: 1 in, 1 out]
        n140 = Enqueue Element(queue=w479, element="element", error in (no error)=w478) -> (error out=w477:errorcluster)  [unwired: 1 in, 2 out]
      }
      event "stop": Value Change {
        n141 = event-data() -> ()  [unwired: 1 in, 1 out]
      }
    }
    n142 = Unbundle By Name(w471) -> ("status"=w470:bool)
    n143 = Or(x=w470, y=w473) -> (x .or. y?=w472:bool)
  }
  n144 = while {
    tunnel: w1 -> [w485]
    stop <- w482 stop-if-true
    # "IO Data (& telemetry analysis?)"
    n145 = Dequeue Element(queue=w485) -> (element=w483:string, error out=w484:errorcluster)  [unwired: 2 in, 2 out]
    n146 = case shown="Error" w484 {
      tunnel: w483 -> [_ _]
      tunnel: [_ TRUE] -> w482
      frame No Error {
        # "Process the data here."
      }
      frame Error {
        # "Return true in any case that should stop the loop."
      }
    }
  }
  n147 = Release Queue(queue=w1, error in (no error)=w3) -> ()  [unwired: 1 in, 3 out]
